vi "Remove last index of path.vi"(11 "Path":path=path "D:/Software/Exe/Data/Plugable Drivers") -> (3 "path":path)   [LabVIEW 2020]
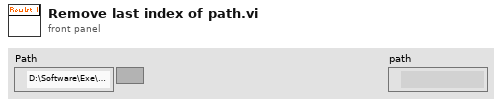
[diagram p1: front panel]
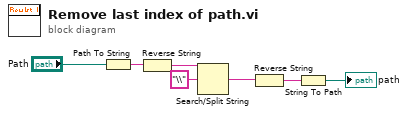
[diagram p0: block diagram]
diagram:
  n1 = Path To String(path="Path") -> (string=w5:string)
  n2 = Reverse String(1:w5) -> (0:w4:string)
  n3 = Search/Split String(string=w4, search string/char (-)="\\") -> (match + rest of string=w3:string)  [unwired: 1 in, 2 out]
  n4 = Reverse String(1:w3) -> (0:w2:string)
  n5 = String To Path(string=w2) -> (path=→"path":path)
